vi "Main Vi.vi"() -> ()   [LabVIEW 2021]
uses:
  <vilib>/Utility/miscctls.llb/LVPointTypeDef.ctl
  <instrlib>/Keithley 2182/Keithley 2182.lvlib
panel:
  in  "Filter Type (0: Moving)":i32(ring)=1 items=["Moving", "Repeat"]
  in  "Polarity reverse mode":bool
  in  "Filter Count (10)":i32=10
  in  "Filter Window (0.01%)":dbl=0.01
  in  "Enable Digital Filter (T: Enable)":bool
  in  "Enable Analog Filter (T: Enable)":bool
  in  "Data Record":bool
  in  "Measurement Interval (ms)":u32=1000
  in  "Measurement Rate":dbl=10.0 min=0.1 max=50.0 format="%#_g PLC"
  in  "Measurement Range":dbl=10.0 format="%#_6p V"
  in  "Auto Range (T: Enable)":bool=TRUE
  out "error out":errorcluster={"status"=TRUE, "code"=-1073807346, "source"="VISA Open in Keithley 2182.lvlib:Initialize.vi->Main Vi.vi"}
  out "Voltage":dbl(graph)
  in  "Stop":bool
  out "Measurement":dbl format="%#_6p"
  out "Measurement Metadata":T1
  in  "Voltage Resolution (8)":i32=8
  in  "Measurement (0: Voltage Channel 1)":T2(ring)
  in  "Integration Rate Units (0: Line Cycles)":enum16{"Line Cycles", "Seconds"}(ring)
  in  "VISA resource name":refnum<visa-resource-name>="COM4"
  # "Measurement Channel"
  # "Measurement Range Setting"
  # "Filters Setting"
  # "Meas. Interval & Recording"
  # "Measurement Rate Setting"
  # "Rate Range : 0.1 to 50 PLC\n0.1 PLC is Fastest\n50 PLC is Slowest"
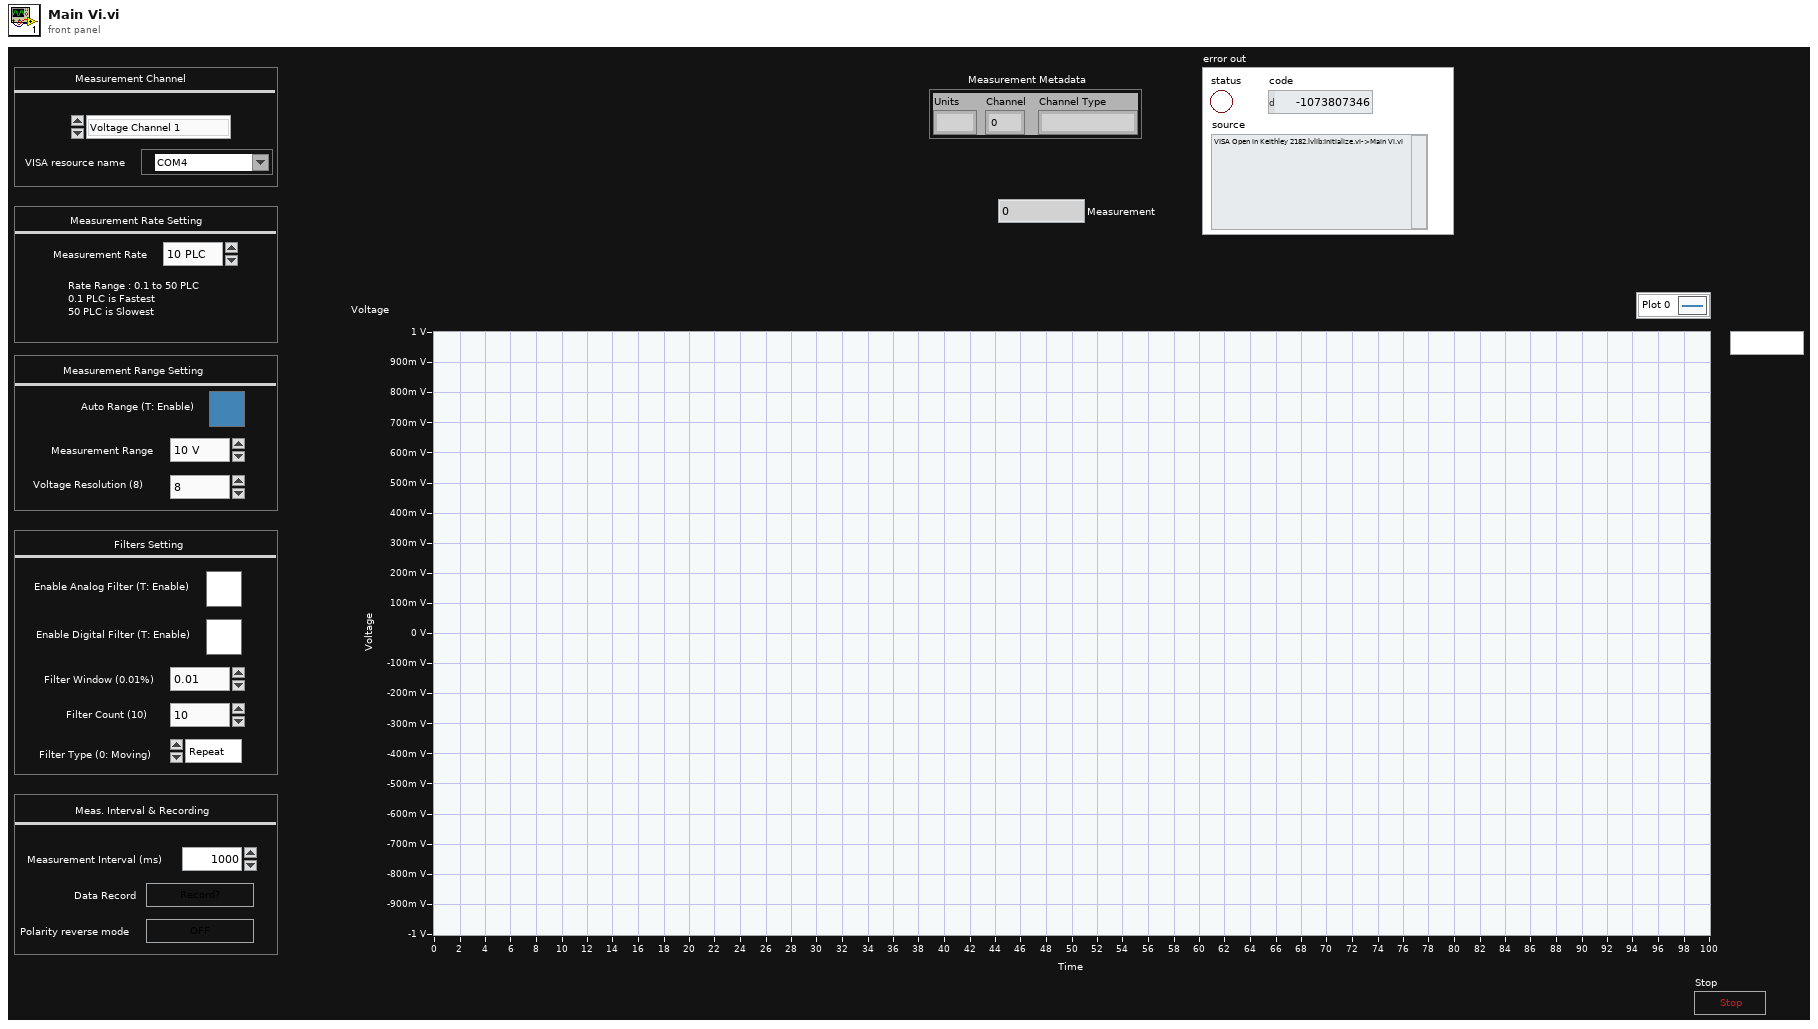
[diagram p1: front panel]
types:
  T1 = cluster{"Units":string, "Channel":i32, "Channel Type":string}
  T2 = enum16{"Voltage Channel 1", "Voltage Channel 2", "Temperature Channel 1", "Temperature Channel 2"}
  T3 = enum16{"open", "open or create", "create or replace", "create", "open (read-only)"}
  T4 = typedef "LVPointTypeDef.ctl" = cluster{"Horizontal":i16, "Vertical":i16}
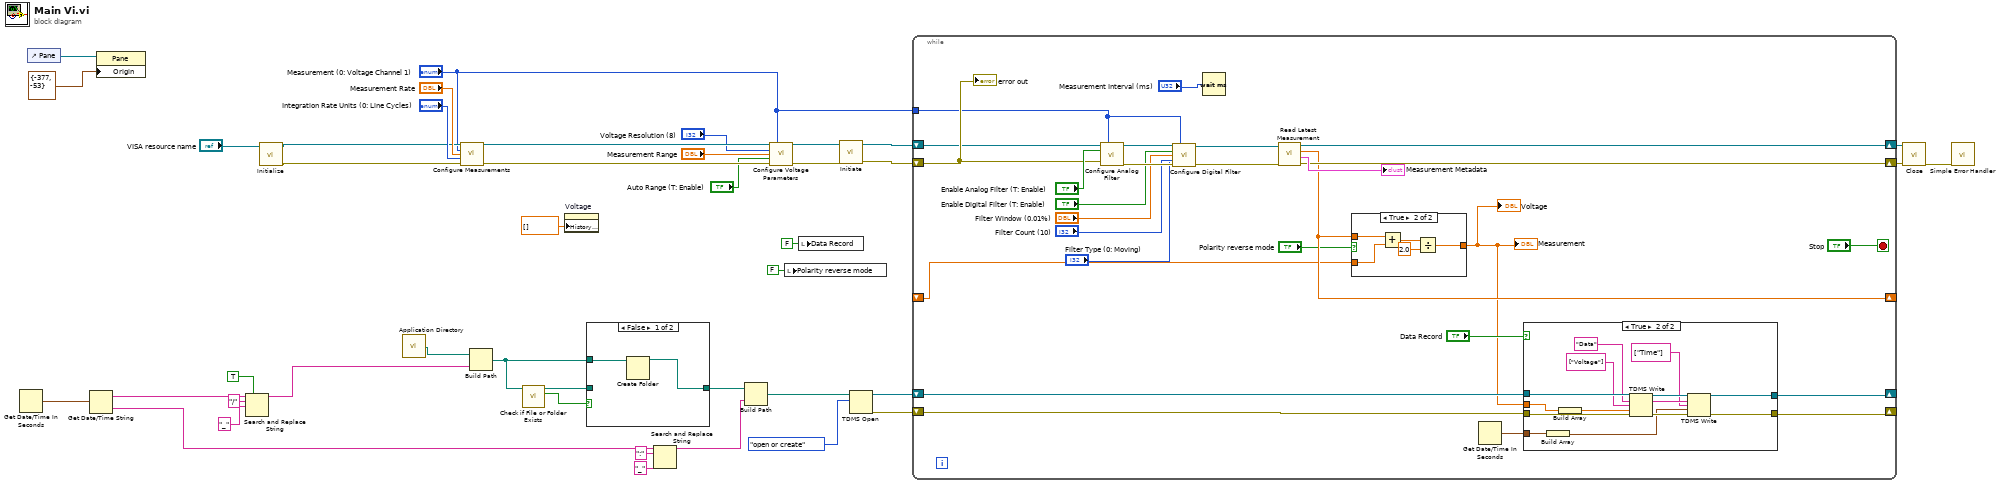
[diagram p0: block diagram]
diagram:
  n1 = Get Date/Time In Seconds() -> (seconds since 1Jan1904=w22:timestamp)
  n2 = control-ref of="Pane"() -> (w24:refnum<vi>)
  n3 = Get Date/Time String(seconds (now)=w22) -> (date string=w21:string, time string=w9:string)  [unwired: 2 in]
  n4 = property class="Pane"(reference=w24, "Origin"=T4 {"Horizontal"=-377, "Vertical"=-53}) -> ()  [unwired: 1 in, 2 out]
  n5 = Search and Replace String(replace all?=TRUE ("replace all? (F)"), input string=w21, search string="/", replace string="_" ("replace string (\"\")")) -> (result string=w16:string)  [unwired: 4 in, 3 out]
  n6 = call <instrlib>:"Initialize.vi"("VISA resource name"="VISA resource name") -> ("error out"=w39:errorcluster, "VISA resource name out"=w38:refnum<visa-resource-name>)  [unwired: 9 in]
  n7 = call <vilib>:"Application Directory.vi"() -> ("Application Directory"=w17:path)
  n8 = call <instrlib>:"Configure Measurements.vi"("VISA resource name"=w38, "Measurement (0: Voltage Channel 1)"="Measurement (0: Voltage Channel 1)", "Integration Rate (5)"="Measurement Rate", "Integration Rate Units (0: Line Cycles)"="Integration Rate Units (0: Line Cycles)", "error in (no error)"=w39) -> ("VISA resource name out"=w36:refnum<visa-resource-name>, "error out"=w37:errorcluster)  [unwired: 9 in]
  n9 = Build Path(base path=w17, name or relative path=w16) -> (appended path=w15:path)
  n10 = call <vilib>:"Check if File or Folder Exists.vi"("path"=w15) -> ("file or folder exists?"=w14:bool, "dup path"=w13:path)  [unwired: 8 in, 1 out]
  n11 = property on="Voltage" class="WFChart (strict)"("History Data"=dbl[] []) -> ()  [unwired: 2 in, 2 out]
  n12 = case shown="False" w14 {
    tunnel: [w44 w45] -> w12
    tunnel: w15 -> [w43 _]
    tunnel: w13 -> [_ w45]
    frame False {
      n13 = Create Folder(path (use dialog)=w43) -> (created path=w44:path)  [unwired: 2 in, 2 out]
    }
    frame True {
    }
  }
  n14 = Search and Replace String(input string=w9, search string=":", replace string="_" ("replace string (\"\")")) -> (result string=w8:string)  [unwired: 5 in, 3 out]
  n15 = Build Path(base path=w12, name or relative path=w8) -> (appended path=w7:path)
  n16 = call <instrlib>:"Configure Voltage Parameters.vi"("VISA resource name"=w36, "Measurement (1: Voltage Channel 1)"="Measurement (0: Voltage Channel 1)", "Voltage Resolution (8)"="Voltage Resolution (8)", "Range Value (12)"="Measurement Range", "Autorange (T: Enable)"="Auto Range (T: Enable)", "error in (no error)"=w37) -> ("VISA resource name out"=w28:refnum<visa-resource-name>, "error out"=w27:errorcluster)  [unwired: 8 in]
  n17 = local write "Polarity reverse mode"(FALSE ("Polarity reverse mode")) -> ()
  n18 = local write "Data Record"(FALSE ("Data Record")) -> ()
  n19 = call <instrlib>:"Initiate.vi"("error in (no error)"=w27, "VISA resource name"=w28) -> ("error out"=w26:errorcluster, "VISA resource name out"=w25:refnum<visa-resource-name>)  [unwired: 8 in]
  n20 = TDMS Open(10:T3."open or create" ("operation (0:open)"), 11:w7) -> (0:w4:errorcluster, 3:w5:refnum<k34>)  [unwired: 5 in]
  n21 = while {
    tunnel: "Measurement (0: Voltage Channel 1)" -> [w62]
    shift-right: [w71] -> w32
    shift-left: w26 -> [w64]
    shift-right: [w70] -> w31
    shift-left: w25 -> [w63]
    shift-right: [w51] -> _
    shift-left: w4 -> [w54]
    shift-right: [w52] -> _
    shift-left: w5 -> [w55]
    shift-right: [w50] -> _
    shift-left: _ -> [w49]
    stop <- "Stop" stop-if-true
    n22 = call <instrlib>:"Configure Analog Filter.vi"("VISA resource name"=w63, "Measurement (0: Voltage Channel 1)"=w62, "Enable Analog Filter (T: Enable)"="Enable Analog Filter (T: Enable)", "error in (no error)"=w64) -> ("VISA resource name out"=w69:refnum<visa-resource-name>, "error out"=w68:errorcluster)  [unwired: 10 in]
    n23 = call <instrlib>:"Configure Digital Filter.vi"("VISA resource name"=w69, "Measurement (0: Voltage Channel 1)"=w62, "Enable Digital Filter (T: Enable)"="Enable Digital Filter (T: Enable)", "Filter Window (0.01%)"="Filter Window (0.01%)", "Filter Count (10)"="Filter Count (10)", "error in (no error)"=w68, "Filter Type (0: Moving)"="Filter Type (0: Moving)") -> ("VISA resource name out"=w67:refnum<visa-resource-name>, "error out"=w66:errorcluster)  [unwired: 7 in]
    n24 = Wait (ms)(milliseconds to wait="Measurement Interval (ms)") -> ()  [unwired: 1 out]
    n25 = call <instrlib>:"Read Latest Measurement.vi"("error in (no error)"=w66, "VISA resource name"=w67) -> ("error out"=w71:errorcluster, "Measurement Metadata"=→"Measurement Metadata":T1, "Measurement"=w50:dbl, "VISA resource name out"=w70:refnum<visa-resource-name>)  [unwired: 6 in]
    n26 = case shown="True" "Polarity reverse mode" {
      tunnel: w50 -> [w73 w78]
      tunnel: w49 -> [_ w77]
      tunnel: [w73 w74] -> w47
      frame False {
      }
      frame True {
        n27 = Add(x=w78, y=w77) -> (x+y=w76:dbl)
        n28 = Divide(x=w76, y=2.0) -> (x/y=w74:dbl)
      }
    }
    "Measurement" <- w47
    "Voltage" <- w47
    n29 = Get Date/Time In Seconds() -> (seconds since 1Jan1904=w53:timestamp)
    n30 = case shown="True" "Data Record" {
      tunnel: w55 -> [w80 w94]
      tunnel: w54 -> [w79 w93]
      tunnel: w47 -> [_ w90]
      tunnel: w53 -> [_ w84]
      tunnel: [w80 w82] -> w52
      tunnel: [w79 w81] -> w51
      frame False {
      }
      frame True {
        n31 = Build Array(w84) -> (w83:timestamp[])
        n32 = Build Array(w90) -> (w89:dbl[])
        n33 = TDMS Write(0:w94, 5:"Data" ("group name in (Untitled)"), 7:string[] ["Voltage"] ("channel name(s) in (Untitled)"), 9:w89, 11:w93) -> (4:w88:refnum<k34>, 6:w86:string, 15:w87:errorcluster)  [unwired: 1 in, 1 out]
        n34 = TDMS Write(0:w88, 5:w86, 7:string[] ["Time"] ("channel name(s) in (Untitled)"), 9:w83, 11:w87) -> (4:w82:refnum<k34>, 15:w81:errorcluster)  [unwired: 1 in, 2 out]
      }
    }
    "error out" <- w64
  }
  n35 = call <instrlib>:"Close.vi"("error in (no error)"=w32, "VISA resource name"=w31) -> ("error out"=w30:errorcluster)  [unwired: 9 in]
  n36 = call <vilib>:"Simple Error Handler.vi"("error in (no error)"=w30) -> ()  [unwired: 4 in, 5 out]
